vi "例5.9   “捆绑”函数.vi"() -> ()   [LabVIEW 2017]
panel:
  out "簇":cluster{string, i32, bool}={"ABC", 1, FALSE}
  out "输出簇 2":cluster{string, i32, bool}
  out "输出簇":cluster{string, i32, bool}
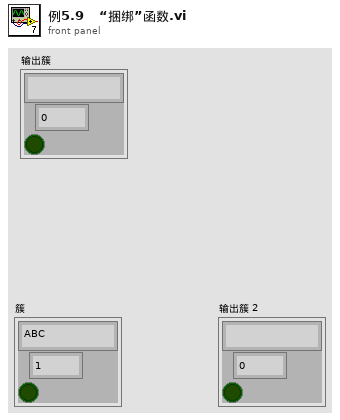
[diagram p1: front panel]
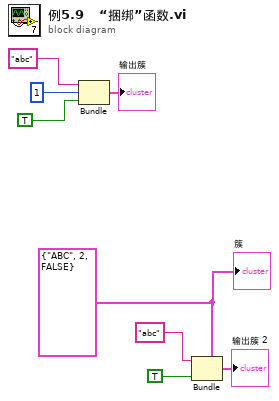
[diagram p0: block diagram]
diagram:
  w1 = cluster{string, i32, bool} {"ABC", 2, FALSE}
  n1 = Bundle("abc", 1, TRUE) -> (→"输出簇":cluster{string, i32, bool})  [unwired: 1 in]
  n2 = Bundle(cluster=w1, "abc", TRUE) -> (→"输出簇 2":cluster{string, i32, bool})  [unwired: 1 in]
  "簇" <- w1
